vi "Read Operation.vi"(0 "Protocols in":refnum<class "Protocols.lvclass">, 11 "Error In":errorcluster) -> (4 "Protocols out":refnum<class "Protocols.lvclass">, 15 "Error Out":errorcluster)   [LabVIEW 2020, in "I2C Controller.lvlib" / "Protocols.lvclass"]
uses:
  Protocols.lvclass
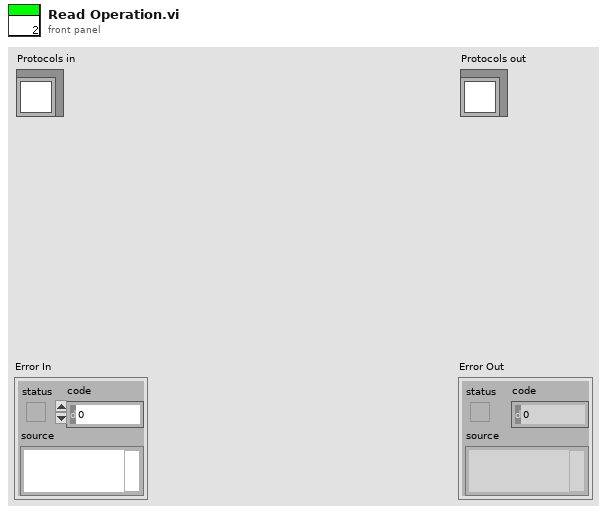
[diagram p1: front panel]
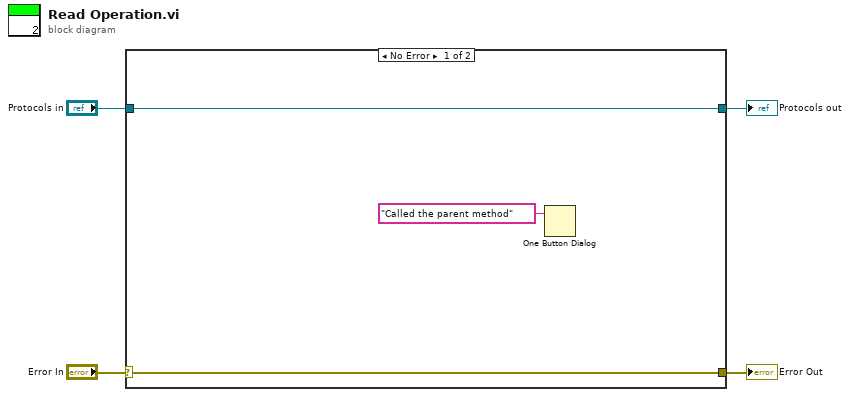
[diagram p0: block diagram]
diagram:
  n1 = case shown="No Error" "Error In" {
    selector: "Error In" -> [w6 w9]
    tunnel: [w6 w9] -> w3
    tunnel: [w7 w8] -> w1
    tunnel: "Protocols in" -> [w7 w8]
    frame No Error {
      n2 = One Button Dialog(message="Called the parent method") -> ()  [unwired: 1 in, 1 out]
    }
    frame Error {
    }
  }
  "Error Out" <- w3
  "Protocols out" <- w1
